vi "N-OrGate.vi"(7 "Stop":bool, 10 "Input":bool) -> (2 "Output":bool)   [LabVIEW 2015]
panel:
  out "Boolean":bool
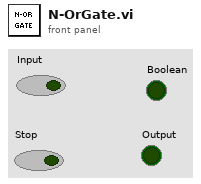
[diagram p1: front panel]
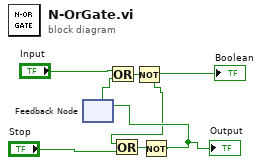
[diagram p0: block diagram]
diagram:
  n1 = feedback #1() -> (w7:bool)  [unwired: 1 in]
  n2 = Or(x="Input", y=w7) -> (x .or. y?=w5:bool)
  n3 = Not(x=w5) -> (.not. x?=w1:bool)
  "Boolean" <- w1
  n4 = Or(x=w1, y="Stop") -> (x .or. y?=w6:bool)
  n5 = Not(x=w6) -> (.not. x?=w4:bool)
  "Output" <- w4
  n6 = feedback-in #1(w4) -> ()
